vi "main OP300.vi"() -> ()   [LabVIEW 2020]
uses:
  <vilib>/Sylvain.lib/02 SLIM ZEN WS 500/SubVi/FGV.ctl
  SubVI/CheminDeBase.vi
  SubVI/OP300ZP_state.ctl
  OP500/VG/VG_progressBar.vi
  VG/IS30%.vi
  VG/PN.vi
  VG/R.vi
  SubVI/VG_HYDRAU.vi
  VG/VG_BT3562.vi
  VG/VG_ST5520.vi
  VG/VG_MX5060.vi
panel:
  out "ISO- avant découpage":string
  out "ISO+":string
  out "ISO-":string
  out "progression":dbl(slide) scale=0.0..60.0
  out "N° Révision":u32
  out "Compt":i32
  in  "DERNIER2":bool
  in  "last?":bool
  out "Cluster 2":T1
  out "IS30% ?":bool
  out "Cluster":T1
  out "VISA OUT":T2
  out "PN":string
  out "errout":errorcluster={"status"=TRUE, "code"=0, "source"="PCAN_CHANNEL ILLEGAL"}
  out "errout":errorcluster caption="sortie d'erreur"
  out "STOP":bool
  out "TOP":string
  out "DRAW":picture
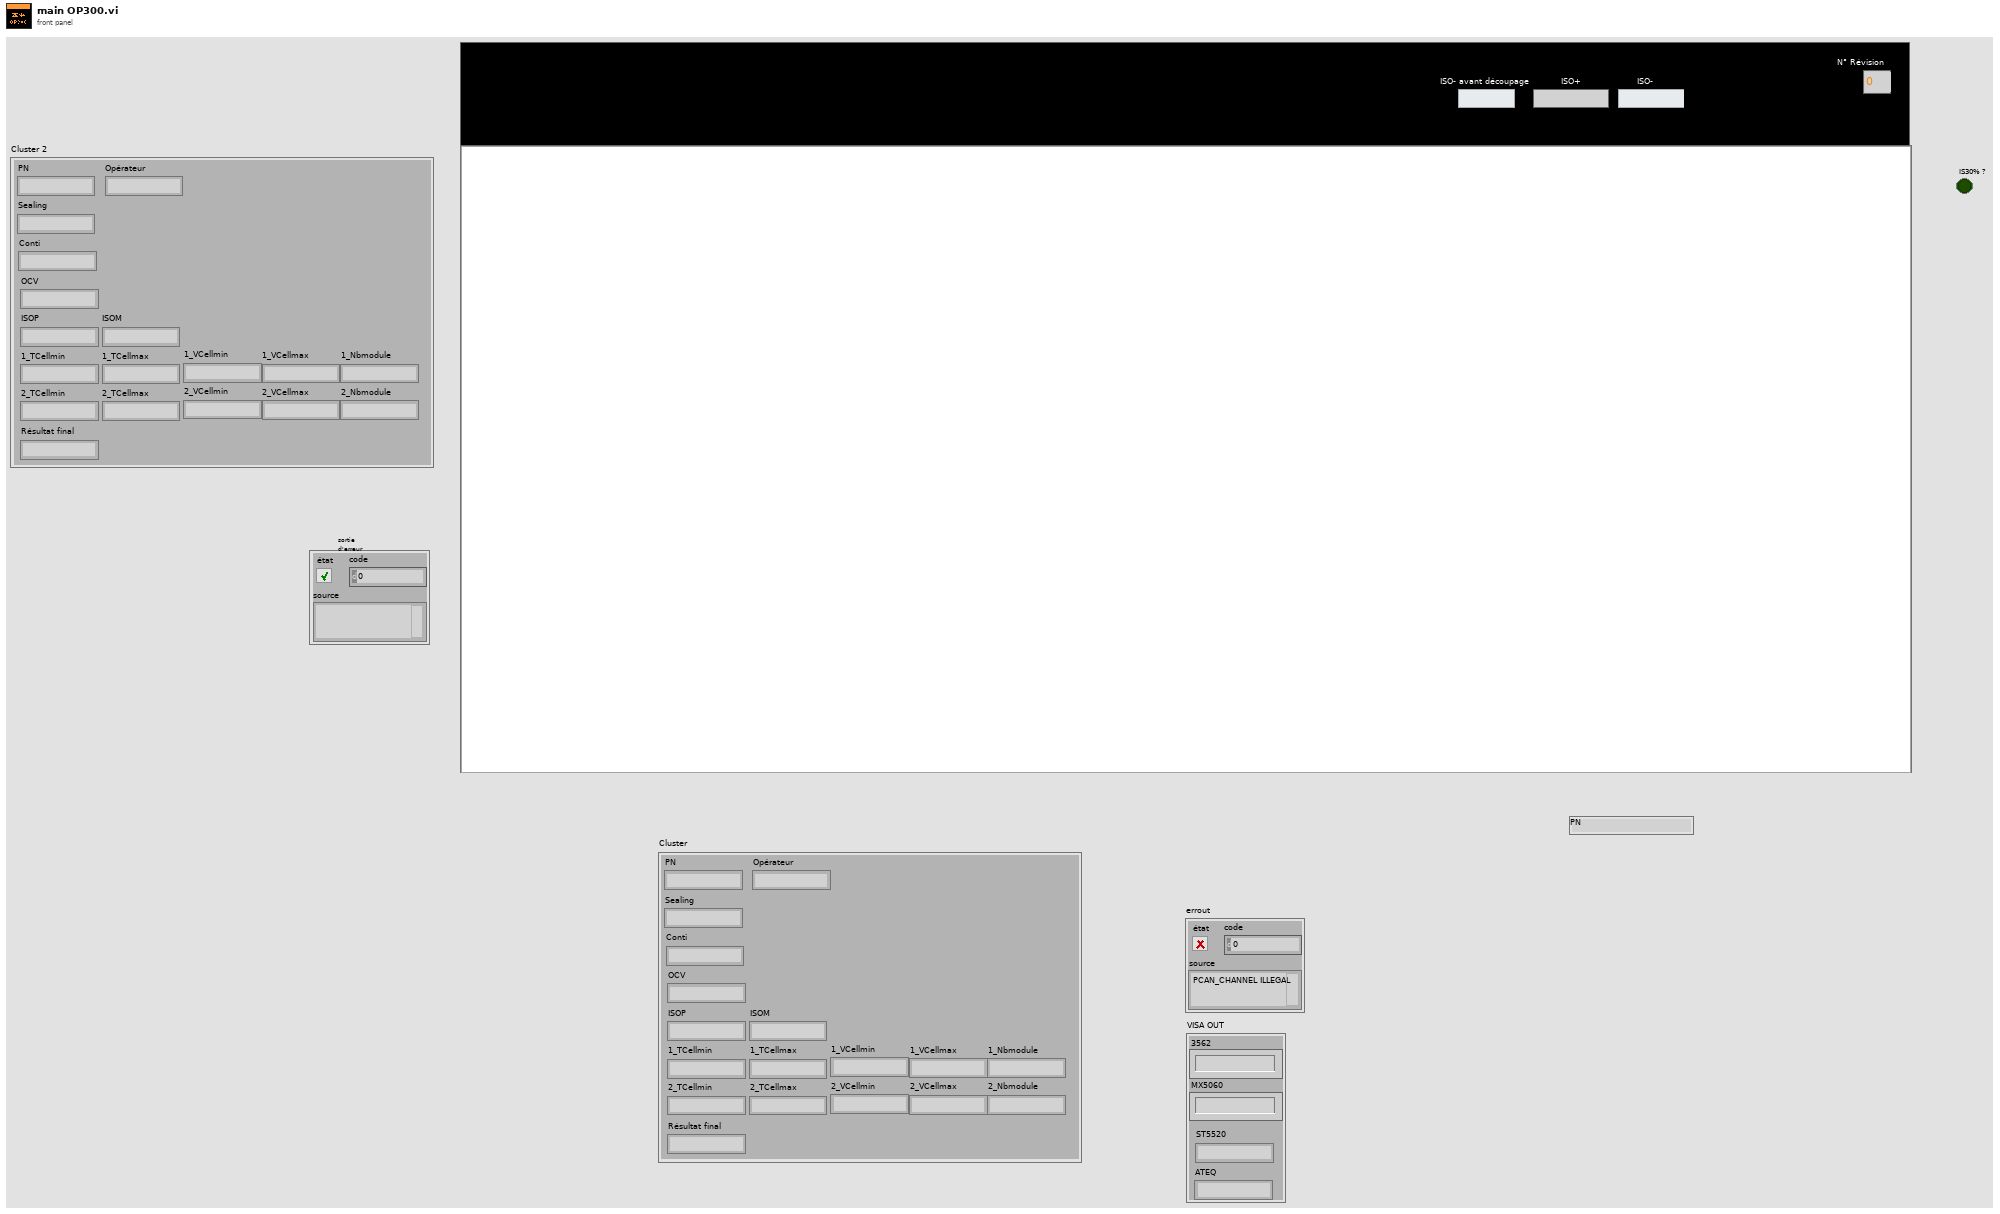
[diagram p1: front panel]
types:
  T1 = cluster{"PN":string, "Opérateur":string, "Sealing":string, "Conti":string, "OCV":string, "ISOP":string, "ISOM":string, "1_TCellmin":string, "1_TCellmax":string, "1_VCellmin":string, "1_VCellmax":string, "1_Nbmodule":string, "2_TCellmin":string, "2_TCellmax":string, "2_VCellmin":string, "2_VCellmax":string, "2_Nbmodule":string, "Résultat final":string}
  T2 = cluster{"3562":string, "MX5060":string, "ST5520":string, "ATEQ":string}
  T3 = cluster{"PN":string, "Sealing":string, "Opérateur":string, "Conti":string, "OCV":string, "ISOP":string, "ISOM":string, "1_TCellmin":string, "1_TCellmax":string, "1_VCellmin":string, "1_VCellmax":string, "1_Nbmodule":string, "2_TCellmin":string, "2_TCellmax":string, "2_VCellmin":string, "2_VCellmax":string, "2_Nbmodule":string, "Résultat final":string}
  T4 = cluster{"3562":string, "MX5060":string, "ST5520":string, "ST5520 2":string}
  T5 = typedef "OP300ZP_state.ctl" = enum16{"Null", "Demarrage", "Init", "Scan", "Montage", "Conti", "OCV", "Iso", "Vpack", "DataDyn", "Dessouter", "DataDyn2", "Demontage", "Crash", "Next", "Hydrau", "Sealing", "Comext"}
  T6 = typedef "FGV.ctl" = enum16{"GET", "SET", "RAZ"}
  T7 = cluster{"1_TCellmin":string, "1_TCellmax":string, "1_VCellmin":string, "1_VCellmax":string, "1_Nbmodule":string, "1_TUsine":string}
  T8 = cluster{"Chaîne":string, "Chaîne":string, "Chaîne":string, "Chaîne":string, "Chaîne":string, "Chaîne":string, "Chaîne":string, "Chaîne 2":string}
  T9 = typedef "imagedata.ctl" = cluster{"image type":i32, "image depth":i32, "image":u8[], "mask":u8[], "colors":u32[], "Rectangle":cluster{"left":i16, "top":i16, "right":i16, "bottom":i16}}
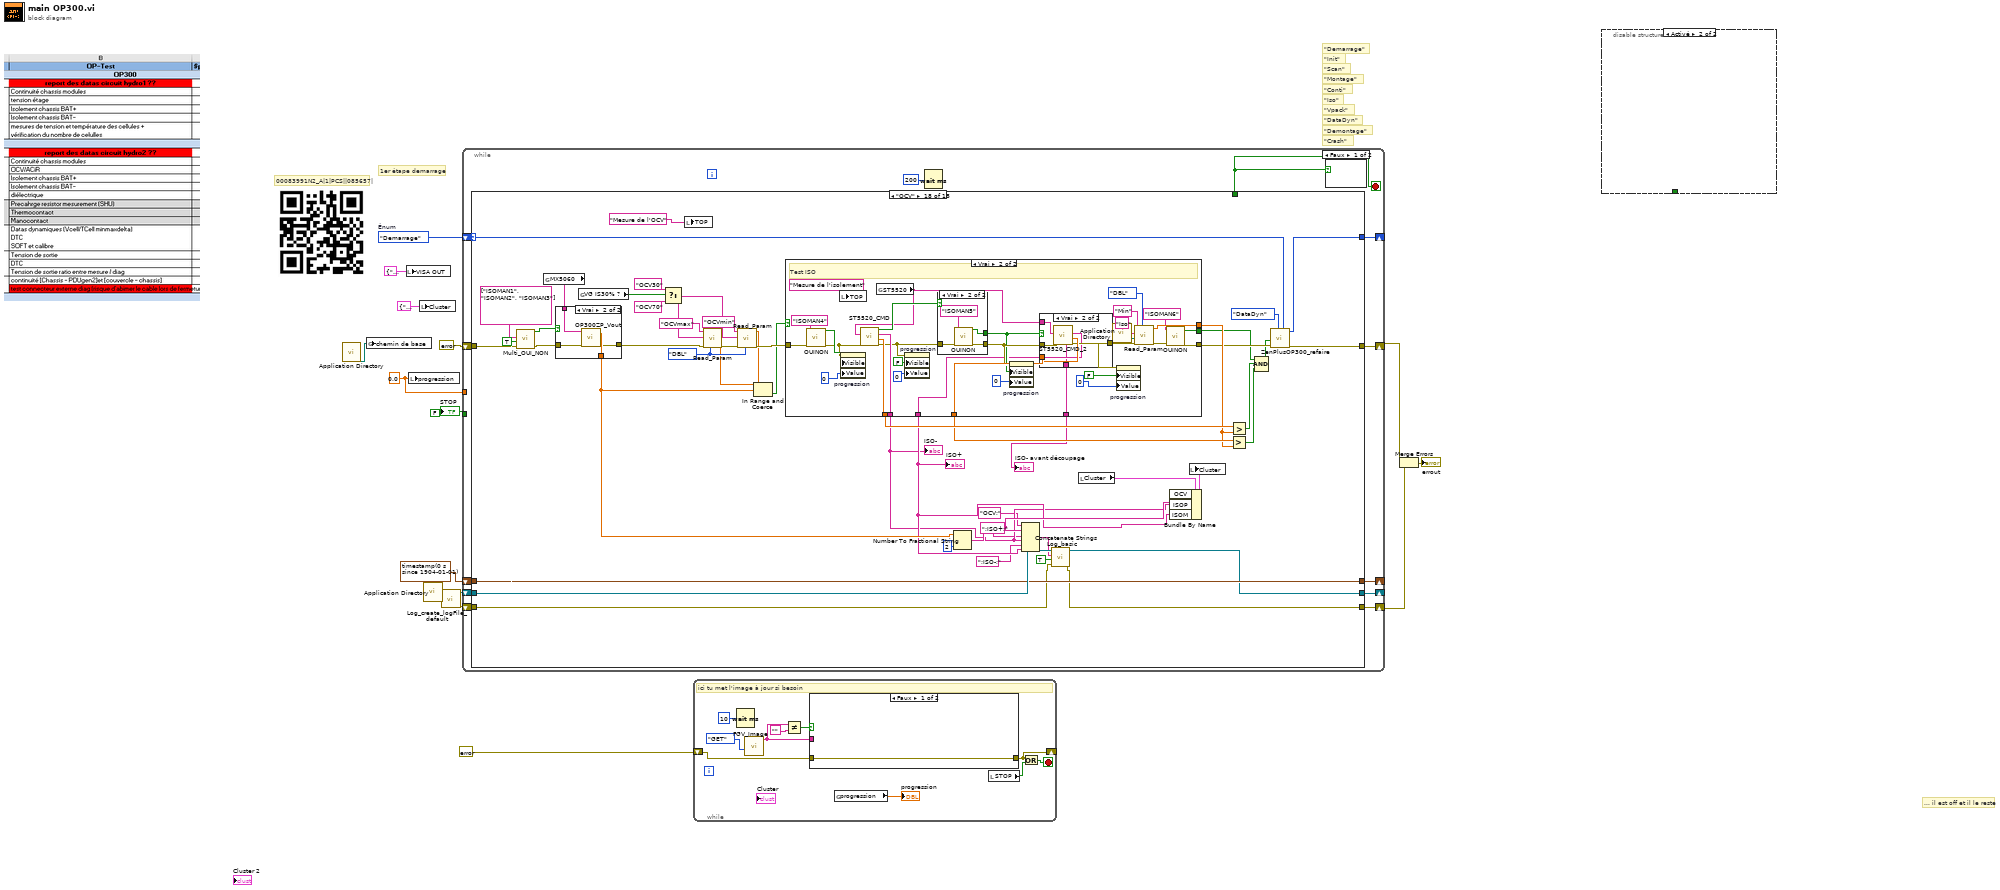
[diagram p0: block diagram]
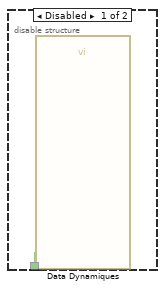
[diagram p2: hidden frame]
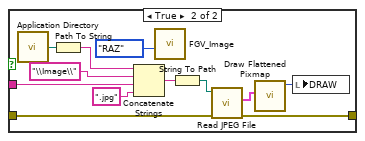
[diagram p3: hidden frame]
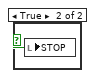
[diagram p4: hidden frame]
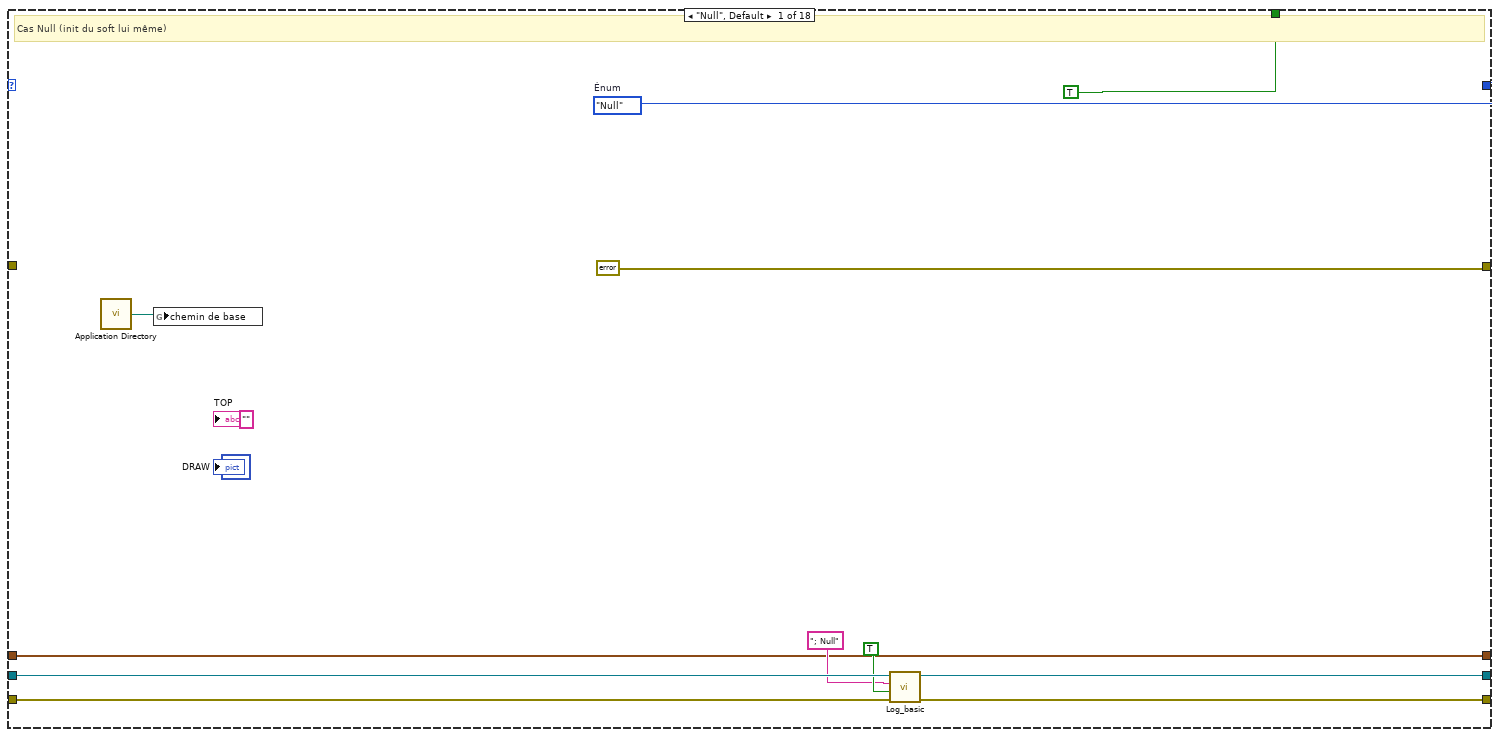
[diagram p5: hidden frame]
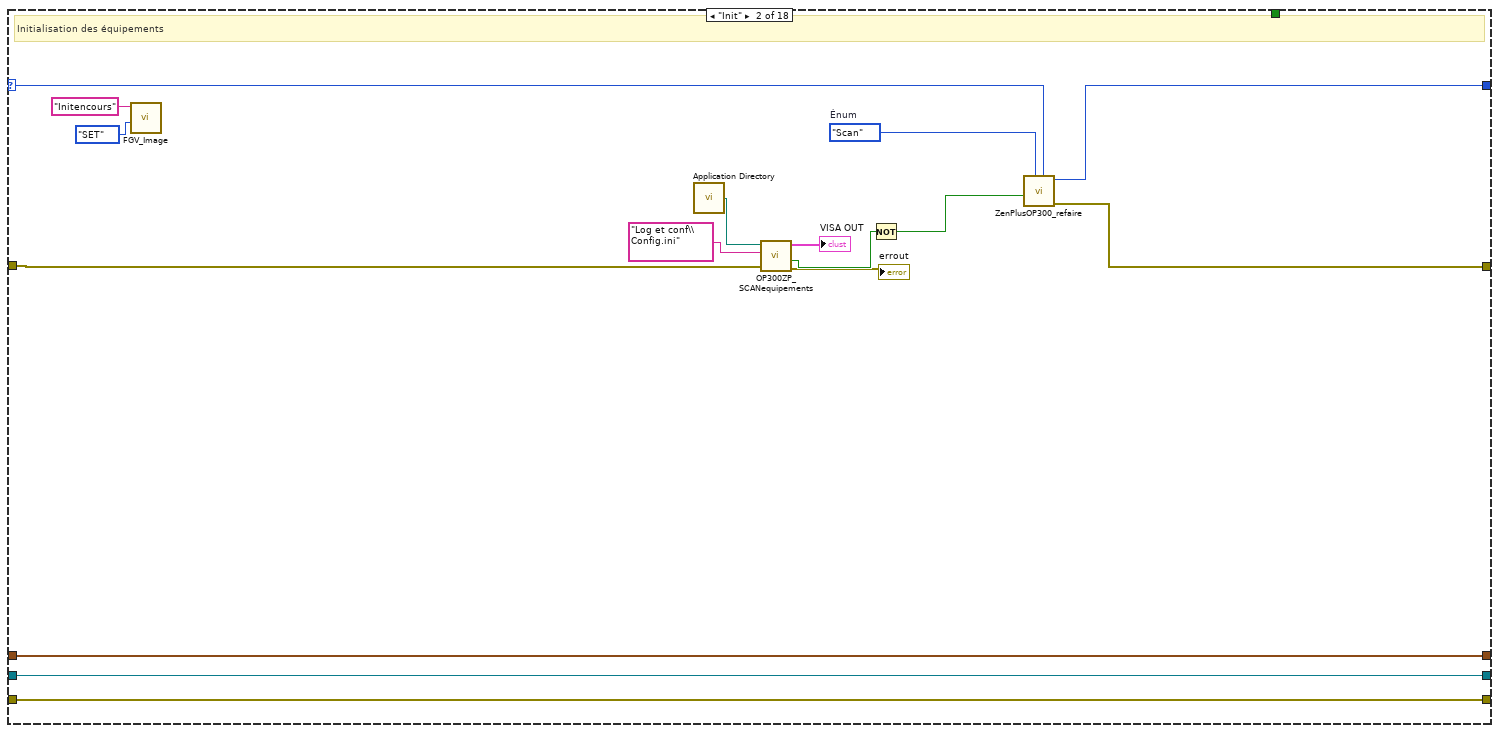
[diagram p6: hidden frame]
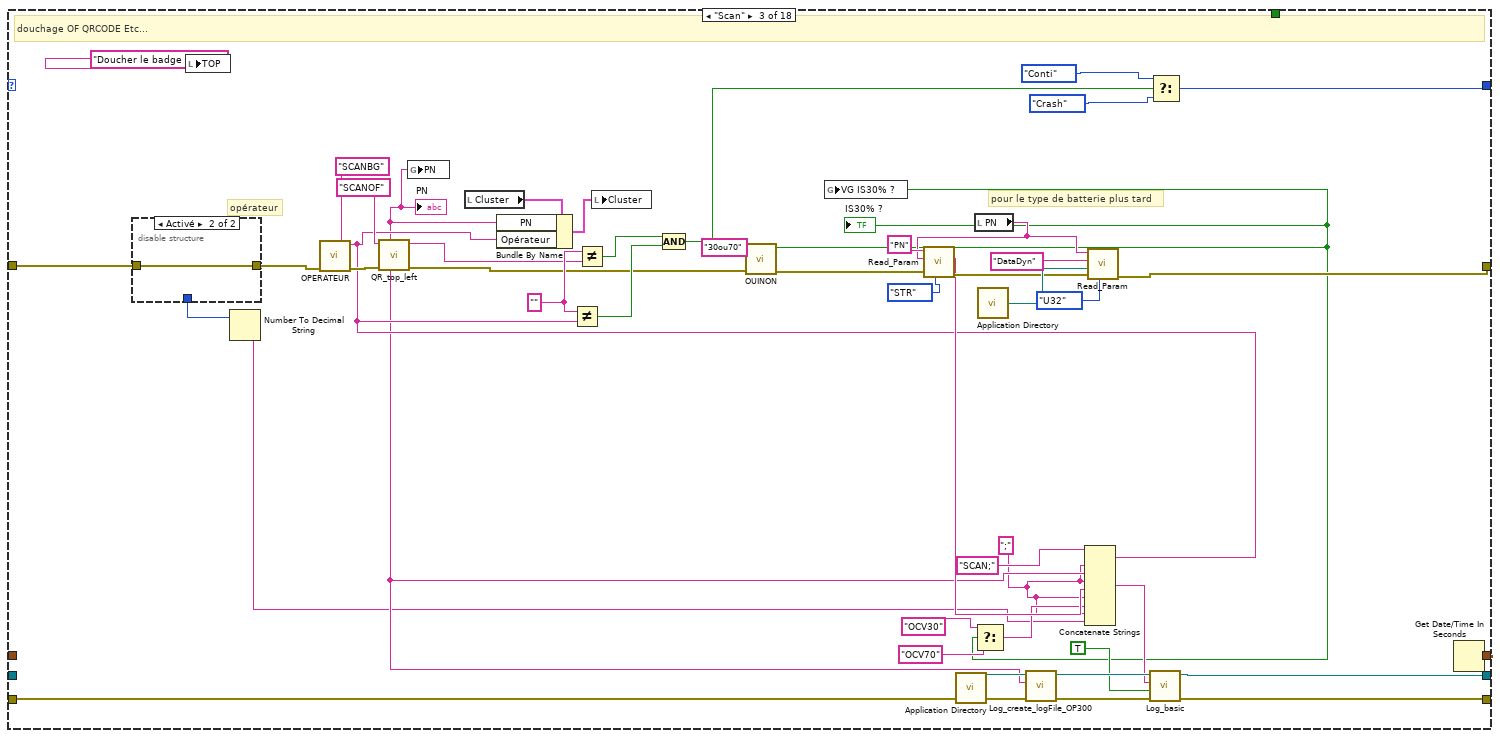
[diagram p7: hidden frame]
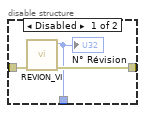
[diagram p8: hidden frame]
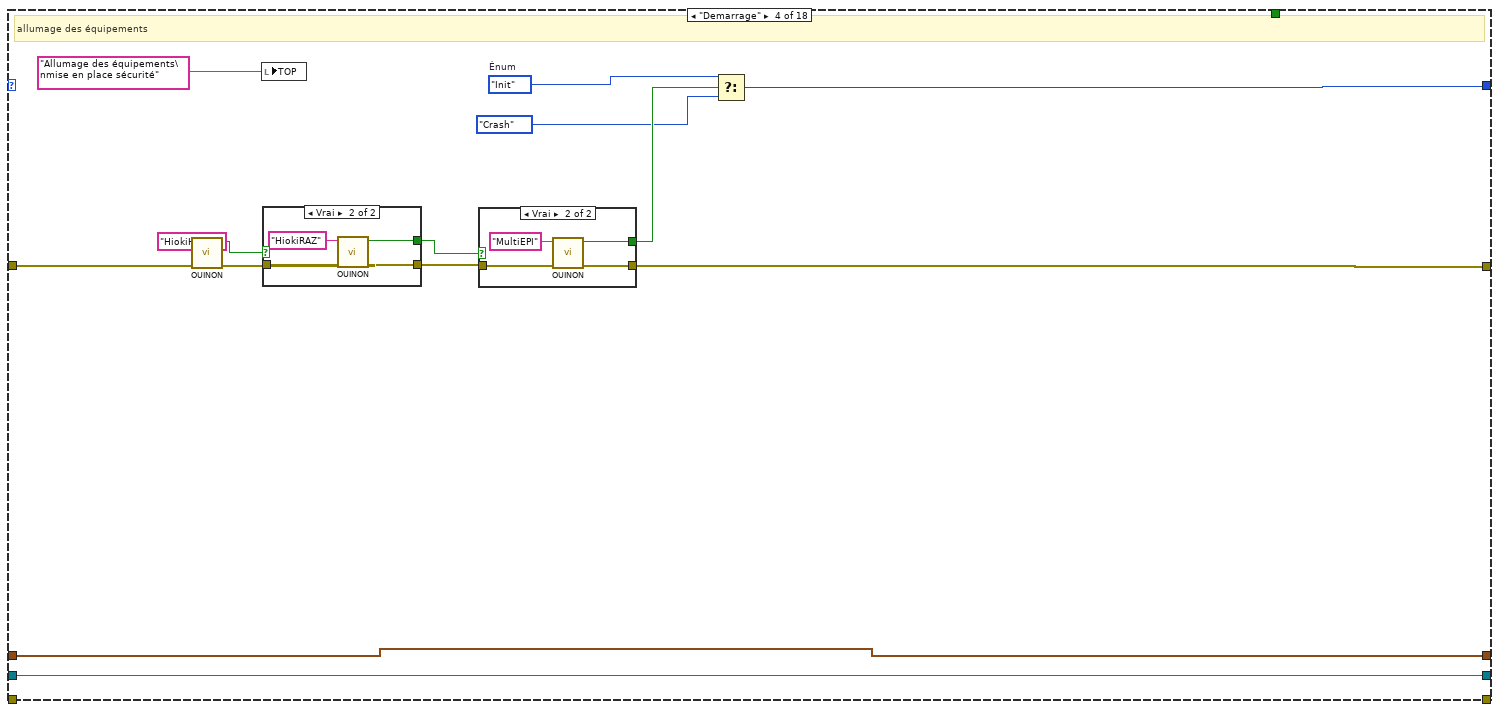
[diagram p9: hidden frame]
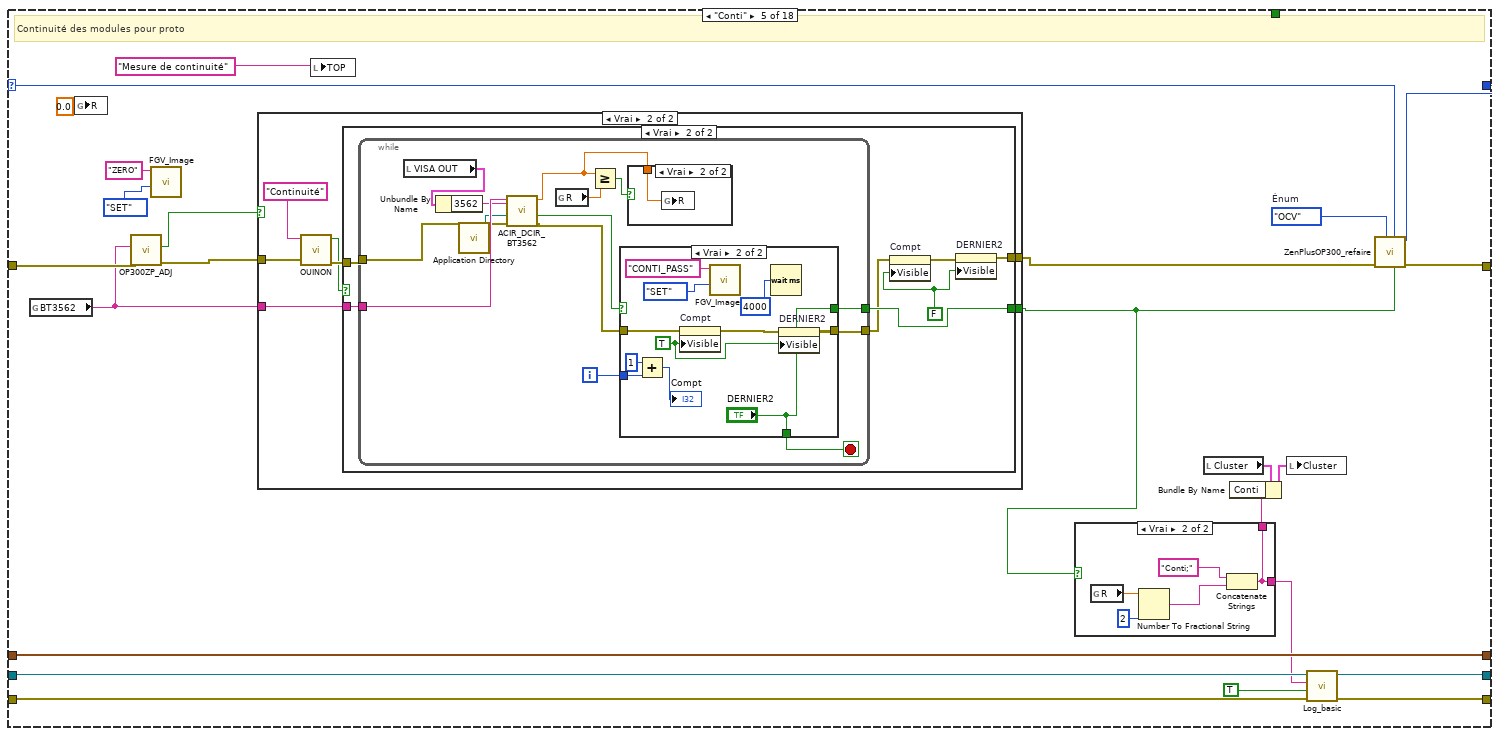
[diagram p12: hidden frame]
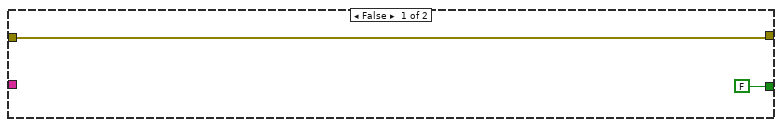
[diagram p13: hidden frame]
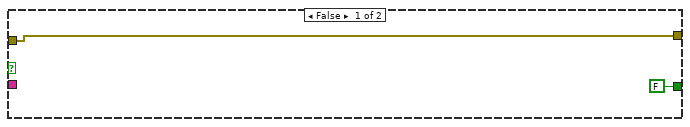
[diagram p14: hidden frame]
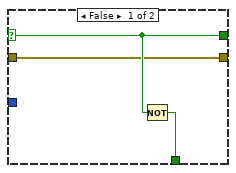
[diagram p15: hidden frame]
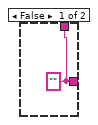
[diagram p17: hidden frame]
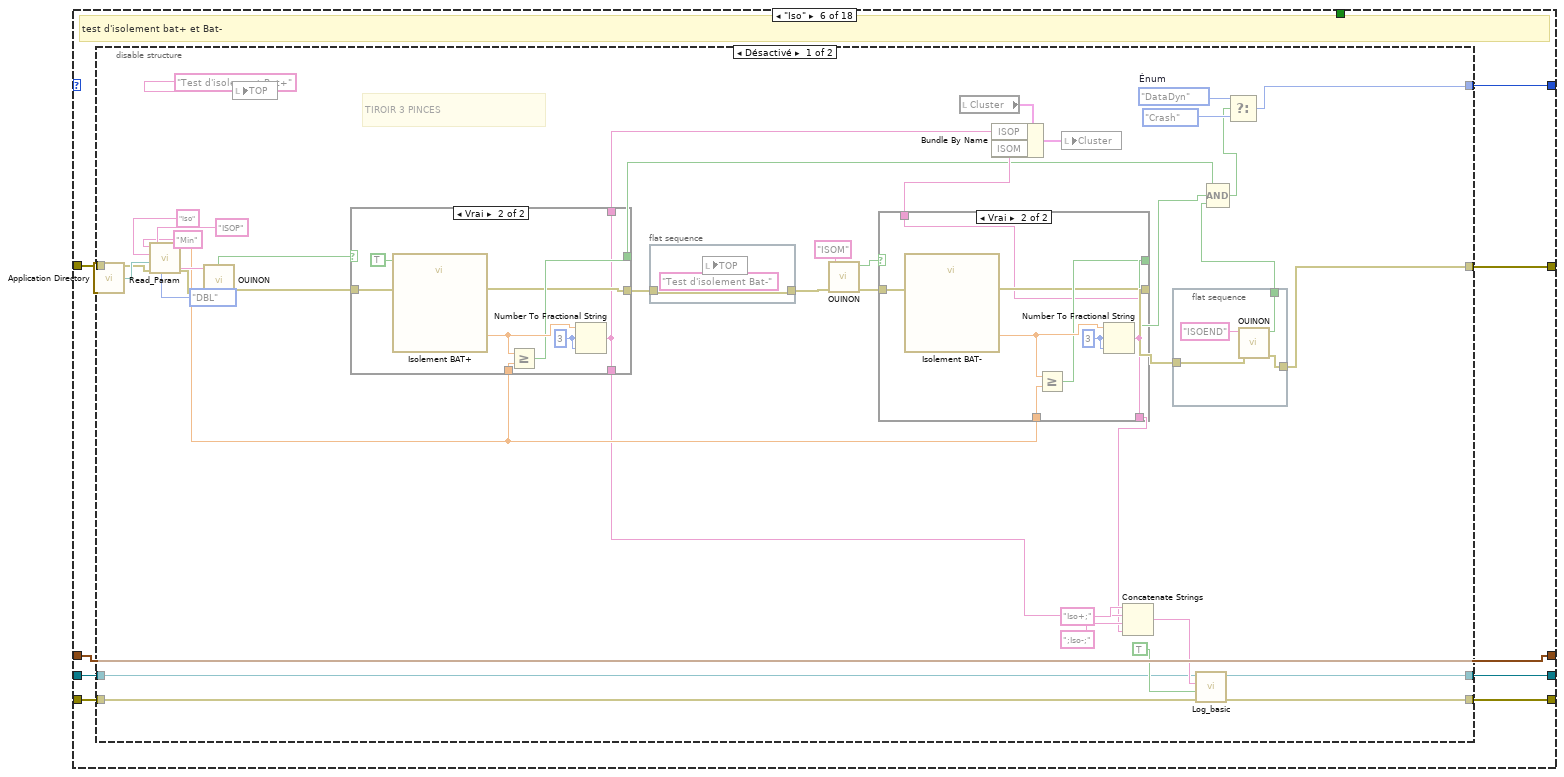
[diagram p18: hidden frame]
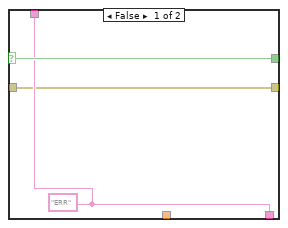
[diagram p19: hidden frame]
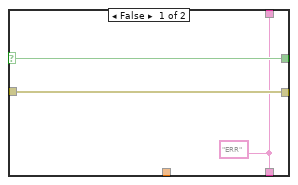
[diagram p20: hidden frame]
diagram:
  w1 = 0.0 ("progression")
  w5 = OP300ZP_state."Demarrage"  # Énum
  w11 = FALSE ("STOP")
  # "00083991N2_A|1|PCS||085657|"
  # "1er étape demarrage"
  # "\"Crash\""
  # "\"Demontage\""
  # "\"DataDyn\""
  # "\"Iso\""
  # "\"Montage\""
  # "\"Scan\""
  # "\"Init\""
  # "\"Demarrage\""
  # "\"Conti\""
  # "\"Vpack\""
  # "... il est off et il le reste"
  n1 = call <vilib>:"Application Directory.vi"() -> ("Application Directory"=w10:path)
  n2 = global write "CheminDeBase.vi" "chemin de base"(w10) -> ()
  n3 = local write "VISA OUT"(T4 {"3562"="", "MX5060"="", "ST5520"="", "ST5520 2"=""} ("VISA OUT")) -> ()
  n4 = local write "progression"(w1) -> ()
  n5 = local write "Cluster"(T3 {"PN"="0", "Sealing"="0", "Opérateur"="0", "Conti"="0", "OCV"="0", "ISOP"="0", "ISOM"="0", "1_TCellmin"="0", "1_TCellmax"="0", "1_VCellmin"="0", "1_VCellmax"="0", "1_Nbmodule"="0", "2_TCellmin"="0", "2_TCellmax"="0", "2_VCellmin"="0", "2_VCellmax"="0", "2_Nbmodule"="0", "Résultat final"="0"} ("Cluster")) -> ()
  n6 = call <vilib>:"Application Directory.vi"() -> ("Application Directory"=w8:path)
  n7 = call <vilib>:"Log_create_logFile_default.vi"("appdir"=w8) -> ("errout"=w9:errorcluster, "Fichier à flux d'octets en sortie"=w12:refnum<file>)  [unwired: 9 in]
  n8 = while {
    shift-right: [w26] -> w14
    shift-left: errorcluster {"status"=FALSE, "code"=0, "source"=""} ("error out") -> [w17]
    shift-right: [w16] -> _
    shift-left: w5 -> [w20]
    shift-right: [w22] -> w13
    shift-left: w9 -> [w25]
    shift-right: [w23] -> _
    shift-left: w12 -> [w24]
    tunnel: w11 -> [_]
    shift-right: [w18] -> _
    shift-left: timestamp(0 s since 1904-01-01) ("seconds since 1Jan1904") -> [w19]
    tunnel: w1 -> [_]
    stop <- w21 stop-if-true
    n9 = case shown="\"OCV\"" w20 {
      selector: w20 -> [_ w53 _ _ w153 _ _ w360 _ w433 _ _ _ _ _ w633 w668 w758]
      tunnel: w17 -> [_ w43 w62 w122 w141 w214 w302 w358 w380 w400 w453 w462 w487 w507 w541 w644 w666 w755]
      tunnel: [errorcluster {"status"=FALSE, "code"=0, "source"=""} ("errin") w54 w86 w121 w154 w215 w306 w359 w387 w395 w452 w461 w487 w505 w544 w631 w667 w763] -> w26
      tunnel: w25 -> [w37 w57 w102 _ w159 w219 w311 w364 w379 w430 w450 w464 w490 w530 w547 w639 w672 w766]
      tunnel: w24 -> [w38 w56 _ w123 w158 w218 w310 w365 w377 w432 w451 w465 w491 w531 w546 w637 w671 w768]
      tunnel: [w35 w56 w104 w123 w157 w217 w309 w362 w377 w428 w451 w465 _ _ w545 w636 w670 w764] -> w23
      tunnel: [w36 w57 w105 _ w156 w220 w308 w363 w379 w429 w450 w464 w480 w523 w542 w638 w669 w765] -> w22
      tunnel: [TRUE _ _ _ _ _ _ _ _ _ _ FALSE w492 _ _ _ _ _] -> w21
      tunnel: w19 -> [w31 w55 _ w120 w155 w216 w289 w361 w378 w431 w449 w460 _ _ w543 w635 w664 w767]
      tunnel: [w31 w55 w93 w120 w155 w216 w289 w361 w378 w431 w449 w460 _ _ w543 w635 w665 w767] -> w18
      tunnel: [w29 w44 w65 w110 w145 w213 w287 w323 w376 w403 w444 w455 OP300ZP_state."Crash" w502 w540 w632 w663 w757] -> w16
      frame "Null", Default {
        w29 = OP300ZP_state."Null"  # Énum
        # "Cas Null (init du soft lui même)"
        n10 = call <vilib>:"Application Directory.vi"() -> ("Application Directory"=w41:path)
        n11 = global write "CheminDeBase.vi" "chemin de base"(w41) -> ()
        n12 = call <vilib>:"Log_basic.vi"("errin"=w37, "date?"=TRUE, "chaîne"="; Null", "in"=w38) -> ("sortie d'erreur"=w36:errorcluster, "refnum en sortie"=w35:refnum<file>)  [unwired: 6 in]
        "DRAW" <- picture data[5B] ("DRAW")
        "TOP" <- "" ("TOP")
      }
      frame "Init" {
        w48 = OP300ZP_state."Scan"  # Énum
        # "Initialisation des équipements"
        n13 = call <vilib>:"FGV_Image.vi"("Énum"=FGV."SET", "IN"="Initencours") -> ()  [unwired: 9 in, 1 out]
        n14 = call <vilib>:"Application Directory.vi"() -> ("Application Directory"=w45:path)
        n15 = call "OP300ZP_SCANequipements.vi"("Errin"=w43, "Chaîne"="Log et conf\\Config.ini", "pathin"=w45) -> ("ERROUT"=→"errout":errorcluster, "KO?"=w49:bool, "VISA OUT"=→"VISA OUT":T2)  [unwired: 6 in]
        n16 = Not(x=w49) -> (.not. x?=w50:bool)
        n17 = call "ZenPlusOP300_refaire.vi"("refaire"=w53, "casOK"=w48, "test ok ?"=w50) -> ("errout"=w54:errorcluster, "Next"=w44:T5)  [unwired: 7 in]
      }
      frame "Scan" {
        w58 = ";" ("chaîne")
        w96 = "" ("x")
        # "pour le type de batterie plus tard"
        # "opérateur"
        # "douchage OF QRCODE Etc..."
        n18 = disable-structure shown="Activé" {
          disable-tunnel: w62 -> [w108 w109]
          disable-tunnel: [w107 w109] -> w61
          disable-tunnel: [w106 _] -> w60
          frame Disabled {
            n19 = call "REVION_VI.vi"("ERRIN"=w108) -> ("ERROUT"=w107:errorcluster, "N° Révision"=w106:u32)  [unwired: 9 in]
            "N° Révision" <- w106
          }
          frame Enabled {
          }
        }
        n20 = local write "TOP"("Doucher le badge et l'OF" ("TOP")) -> ()
        n21 = Number To Decimal String(number=w60) -> (decimal integer string=w59:string)  [unwired: 1 in]
        n22 = call <vilib>:"OPERATEUR.vi"("errin"=w61, "IN"="SCANBG") -> ("error out"=w92:errorcluster, "Dataout"=w73:string)  [unwired: 8 in]
        n23 = call <vilib>:"QR_top_left.vi"("errin"=w92, "image"="SCANOF") -> ("error out"=w63:errorcluster, "Réponse"=w90:string, "SN"=w64:string, "PN"=w66:string)  [unwired: 5 in, 1 out]
        "PN" <- w66
        n24 = global write "PN.vi" "PN"(w66) -> ()
        n25 = local read "Cluster"() -> (w75:T1)
        n26 = Bundle By Name(cluster=w75, "PN"=w66, "Opérateur"=w73) -> (w74:T1)
        n27 = Not Equal?(x=w96, y=w73) -> (x != y?=w94:bool)
        n28 = Not Equal?(x=w96, y=w90) -> (x != y?=w95:bool)
        n29 = local write "Cluster"(w74) -> ()
        n30 = Compound Arithmetic op=AND ("Opérateur arithmétique")(w95, w94) -> (w79:bool)
        n31 = call <vilib>:"OUINON.vi"("errin"=w63, "image"="30ou70") -> ("error out"=w71:errorcluster, "OUI/NON"=w67:bool)  [unwired: 8 in]
        "IS30% ?" <- w67
        n32 = global write "IS30%.vi" "VG IS30% ?"(w67) -> ()
        n33 = call <vilib>:"Application Directory.vi"() -> ("Application Directory"=w103:path)
        n34 = local read "PN"() -> (w82:string)
        n35 = call "Read_Param.vi"("Énum"=enum16{"STR", "DBL", "U32"}."STR", "errin"=w71, "section"=w82, "key"="PN") -> ("error out"=w85:errorcluster, "str"=w81:string)  [unwired: 3 in, 3 out]
        n36 = Select ("Sélectionner")(t="OCV30" ("section"), s=w67, f="OCV70" ("section")) -> (s? t:f=w68:string)
        n37 = call <vilib>:"Application Directory.vi"() -> ("Application Directory"=w89:path)
        n38 = call "Log_create_logFile_OP300.vi"("errin"=w102, "toute l'expression"=w64, "Application Directory"=w103) -> ("sortie d'erreur"=w100:errorcluster, "Fichier à flux d'octets en sortie"=w101:refnum<file>)  [unwired: 7 in]
        n39 = Concatenate Strings("SCAN;" ("chaîne"), w73, w58, w64, w58, w81, w58, w68, w58, w59) -> (w98:string)
        n40 = call "Read_Param.vi"("Énum"=enum16{"STR", "DBL", "U32"}."U32", "errin"=w85, 9:w89, "section"="DataDyn", "key"=w82) -> ("error out"=w86:errorcluster)  [unwired: 2 in, 4 out]
        n41 = call <vilib>:"Log_basic.vi"("errin"=w100, "date?"=TRUE, "chaîne"=w98, "in"=w101) -> ("sortie d'erreur"=w105:errorcluster, "refnum en sortie"=w104:refnum<file>)  [unwired: 6 in]
        n42 = Select ("Sélectionner")(t=OP300ZP_state."Conti" ("Énum"), s=w79, f=OP300ZP_state."Crash" ("cas faux")) -> (s? t:f=w65:T5)
        n43 = Get Date/Time In Seconds() -> (seconds since 1Jan1904=w93:timestamp)
      }
      frame "Demarrage" {
        w112 = OP300ZP_state."Init"  # Énum
        # "allumage des équipements"
        n44 = call <vilib>:"OUINON.vi"("errin"=w122, "image"="HiokiHypot") -> ("error out"=w118:errorcluster, "OUI/NON"=w115:bool)  [unwired: 8 in]
        n45 = local write "TOP"("Allumage des équipements\nmise en place sécurité" ("TOP")) -> ()
        n46 = case shown="Vrai" w115 {
          selector: w115 -> [w125 _]
          tunnel: [w125 w129] -> w116
          tunnel: [w124 w128] -> w117
          tunnel: w118 -> [w124 w126]
          frame False {
          }
          frame True {
            n47 = call <vilib>:"OUINON.vi"("errin"=w126, "image"="HiokiRAZ" ("IN")) -> ("error out"=w128:errorcluster, "OUI/NON"=w129:bool)  [unwired: 8 in]
          }
        }
        n48 = case shown="Vrai" w116 {
          selector: w116 -> [w131 _]
          tunnel: [w131 w135] -> w113
          tunnel: [w130 w134] -> w121
          tunnel: w117 -> [w130 w132]
          frame False {
          }
          frame True {
            n49 = call <vilib>:"OUINON.vi"("errin"=w132, "image"="MultiEPI" ("IN")) -> ("error out"=w134:errorcluster, "OUI/NON"=w135:bool)  [unwired: 8 in]
          }
        }
        n50 = Select ("Sélectionner")(t=w112, s=w113, f=OP300ZP_state."Crash" ("cas faux")) -> (s? t:f=w110:T5)
      }
      frame "Conti" {
        w149 = OP300ZP_state."OCV"  # Énum
        # "Continuité des modules pour proto"
        n51 = global read "VG_BT3562.vi" "BT3562"() -> (w137:string)
        n52 = global write "R.vi" "R"(0.0 ("R")) -> ()
        n53 = call "OP300ZP_ADJ.vi"("errin"=w141, "BT3562A"=w137) -> ("errout"=w140:errorcluster, "ADJ?"=w138:bool)  [unwired: 8 in]
        n54 = call <vilib>:"FGV_Image.vi"("Énum"=FGV."SET", "IN"="ZERO") -> ()  [unwired: 9 in, 1 out]
        n55 = case shown="Vrai" w138 {
          tunnel: [FALSE ("DERNIER2") w168] -> w146
          tunnel: [w161 w167] -> w147
          tunnel: w140 -> [w161 w164]
          tunnel: w137 -> [_ w166]
          frame False {
          }
          frame True {
            n56 = call <vilib>:"OUINON.vi"("errin"=w164, "image"="Continuité" ("IN")) -> ("error out"=w163:errorcluster, "OUI/NON"=w162:bool)  [unwired: 8 in]
            n57 = case shown="Vrai" w162 {
              tunnel: [FALSE ("DERNIER2") w177] -> w168
              tunnel: [w170 w176] -> w167
              tunnel: w166 -> [_ w172]
              tunnel: w163 -> [w170 w171]
              frame False {
              }
              frame True {
                w173 = FALSE ("Visible")
                n58 = while {
                  tunnel: w172 -> [w191]
                  tunnel: w171 -> [w190]
                  tunnel: [w187] -> w175
                  tunnel: [w182] -> w177
                  i -> [w186]
                  stop <- w181 stop-if-true
                  n59 = local read "VISA OUT"() -> (w179:T2)
                  n60 = Unbundle By Name(w179) -> ("3562"=w178:string)
                  n61 = call <vilib>:"Application Directory.vi"() -> ("Application Directory"=w189:path)
                  n62 = call <userlib>:"ACIR_DCIR_BT3562.vi"("errin"=w190, "chemin de base"=w189, "section"=w178, "VISAin"=w191) -> ("errout"=w180:errorcluster, "R pass"=w188:bool, "R Out float"=w183:dbl)  [unwired: 1 in, 4 out]
                  n63 = global read "R.vi" "R"() -> (w185:dbl)
                  n64 = Greater Or Equal?(x=w183, y=w185) -> (x >= y?=w184:bool)
                  n65 = case shown="Vrai" w188 {
                    selector: w188 -> [w194 _]
                    tunnel: w180 -> [w192 w201]
                    tunnel: [w192 w197] -> w187
                    tunnel: [w193 "DERNIER2"] -> w181
                    tunnel: w186 -> [_ w203]
                    tunnel: [w194 "DERNIER2"] -> w182
                    frame False {
                      n66 = Not(x=w194) -> (.not. x?=w193:bool)
                    }
                    frame True {
                      w195 = TRUE ("Visible")
                      n67 = Add(x=1, y=w203) -> (x+y=→"Compt":i32)
                      n68 = property on="Compt" class="NumNb (strict)"(error in=w201, "Visible"=w195) -> (error out=w198:errorcluster)  [unwired: 1 in, 1 out]
                      n69 = call <vilib>:"FGV_Image.vi"("Énum"=FGV."SET", "IN"="CONTI_PASS") -> ()  [unwired: 9 in, 1 out]
                      n70 = Wait (ms)(milliseconds to wait=u32 4000 ("attente (ms)")) -> ()  [unwired: 1 out]
                      n71 = property on="DERNIER2" class="Bool"(error in=w198, "Visible"=w195) -> (error out=w197:errorcluster)  [unwired: 1 in, 1 out]
                    }
                  }
                  n72 = case shown="Vrai" w184 {
                    tunnel: w183 -> [_ w206]
                    frame False {
                    }
                    frame True {
                      n73 = global write "R.vi" "R"(w206) -> ()
                    }
                  }
                }
                n74 = property on="Compt" class="NumNb (strict)"(error in=w175, "Visible"=w173) -> (error out=w174:errorcluster)  [unwired: 1 in, 1 out]
                n75 = property on="DERNIER2" class="Bool"(error in=w174, "Visible"=w173) -> (error out=w176:errorcluster)  [unwired: 1 in, 1 out]
              }
            }
          }
        }
        n76 = local write "TOP"("Mesure de continuité" ("TOP")) -> ()
        n77 = case shown="Vrai" w146 {
          tunnel: [w207 w208] -> w152
          tunnel: [w207 w208] -> w142
          frame False {
            w207 = ""
          }
          frame True {
            n78 = global read "R.vi" "R"() -> (w211:dbl)
            n79 = Number To Fractional String(number=w211, precision (6)=i16 2 ("précision (6)")) -> (F-format string=w210:string)  [unwired: 2 in]
            n80 = Concatenate Strings("Conti;" ("chaîne"), w210) -> (w208:string)
          }
        }
        n81 = local read "Cluster"() -> (w144:T1)
        n82 = Bundle By Name(cluster=w144, "Conti"=w142) -> (w143:T1)
        n83 = local write "Cluster"(w143) -> ()
        n84 = call <vilib>:"Log_basic.vi"("errin"=w159, "date?"=TRUE, "chaîne"=w152, "in"=w158) -> ("sortie d'erreur"=w156:errorcluster, "refnum en sortie"=w157:refnum<file>)  [unwired: 6 in]
        n85 = call "ZenPlusOP300_refaire.vi"("refaire"=w153, "casOK"=w149, "errin"=w147, "test ok ?"=w146) -> ("errout"=w154:errorcluster, "Next"=w145:T5)  [unwired: 6 in]
      }
      frame "Iso" {
        # "test d'isolement bat+ et Bat-"
        n86 = disable-structure shown="Désactivé" {
          disable-tunnel: [w247 _] -> w220
          disable-tunnel: w219 -> [w246 _]
          disable-tunnel: w218 -> [w245 _]
          disable-tunnel: [w244 _] -> w217
          disable-tunnel: [w234 _] -> w215
          disable-tunnel: w214 -> [w222 _]
          disable-tunnel: [w221 _] -> w213
          frame Disabled {
            w240 = OP300ZP_state."DataDyn"  # Énum
            # "TIROIR 3 PINCES"
            n87 = call <vilib>:"Application Directory.vi"() -> ("Application Directory"=w255:path)
            n88 = call "Read_Param.vi"("Énum"=enum16{"STR", "DBL", "U32"}."DBL", "errin"=w222, 9:w255, "section"="Iso", "key"="Min") -> ("error out"=w252:errorcluster, "dbl"=w249:dbl)  [unwired: 2 in, 3 out]
            n89 = call <vilib>:"OUINON.vi"("errin"=w252, "image"="ISOP" ("IN")) -> ("error out"=w227:errorcluster, "OUI/NON"=w228:bool)  [unwired: 8 in]
            n90 = local write "TOP"("Test d'isolement Bat+" ("TOP")) -> ()
            n91 = case shown="Vrai" w228 {
              selector: w228 -> [w277 _]
              tunnel: w227 -> [w278 w286]
              tunnel: [w278 w281] -> w225
              tunnel: [w276 w280] -> w242
              tunnel: [w277 w282] -> w232
              tunnel: w249 -> [_ w284]
              tunnel: [w276 w280] -> w236
              frame False {
                w276 = "ERR"
              }
              frame True {
                w285 = i16 3 ("largeur (-)")
                n92 = call "Isolement BAT+"("Enable"=TRUE, "error in (no error)"=w286) -> ("ISOP"=w283:dbl, "error out"=w281:errorcluster)  [unwired: 15 in, 1 out]
                n93 = Greater Or Equal?(x=w283, y=w284) -> (x >= y?=w282:bool)
                n94 = Number To Fractional String(number=w283, width (-)=w285, precision (6)=w285) -> (F-format string=w280:string)  [unwired: 1 in]
              }
            }
            n95 = flat-sequence {
              tunnel: w225 -> [w260]
              tunnel: [w260] -> w224
              frame #0 {
                n96 = local write "TOP"("Test d'isolement Bat-" ("TOP")) -> ()
              }
            }
            n97 = call <vilib>:"OUINON.vi"("errin"=w224, "image"="ISOM" ("IN")) -> ("error out"=w226:errorcluster, "OUI/NON"=w250:bool)  [unwired: 8 in]
            n98 = case shown="Vrai" w250 {
              selector: w250 -> [w268 _]
              tunnel: [w266 w271] -> w233
              tunnel: [w267 w270] -> w241
              tunnel: [w268 w272] -> w231
              tunnel: w249 -> [_ w274]
              tunnel: [w267 w270] -> w235
              tunnel: w226 -> [w266 w269]
              frame False {
                w267 = "ERR"
              }
              frame True {
                w275 = i16 3 ("largeur (-)")
                n99 = call "Isolement BAT-"("error in (no error)"=w269) -> ("ISOM"=w273:dbl, "error out"=w271:errorcluster)  [unwired: 16 in, 1 out]
                n100 = Greater Or Equal?(x=w273, y=w274) -> (x >= y?=w272:bool)
                n101 = Number To Fractional String(number=w273, width (-)=w275, precision (6)=w275) -> (F-format string=w270:string)  [unwired: 1 in]
              }
            }
            n102 = local read "Cluster"() -> (w238:T1)
            n103 = Bundle By Name(cluster=w238, "ISOP"=w236, "ISOM"=w235) -> (w237:T1)
            n104 = local write "Cluster"(w237) -> ()
            n105 = Concatenate Strings("Iso+;" ("chaîne"), w242, ";Iso-;" ("chaîne"), w241) -> (w258:string)
            n106 = flat-sequence {
              tunnel: [w263] -> w234
              tunnel: w233 -> [w264]
              tunnel: [w262] -> w230
              frame #0 {
                n107 = call <vilib>:"OUINON.vi"("errin"=w264, "image"="ISOEND") -> ("error out"=w263:errorcluster, "OUI/NON"=w262:bool)  [unwired: 8 in]
              }
            }
            n108 = call <vilib>:"Log_basic.vi"("errin"=w246, "date?"=TRUE, "chaîne"=w258, "in"=w245) -> ("sortie d'erreur"=w247:errorcluster, "refnum en sortie"=w244:refnum<file>)  [unwired: 6 in]
            n109 = Compound Arithmetic op=AND ("Opérateur arithmétique")(w232, w231, w230) -> (w229:bool)
            n110 = Select ("Sélectionner")(t=w240, s=w229, f=OP300ZP_state."Crash" ("cas faux")) -> (s? t:f=w221:T5)
          }
          frame Enabled {
          }
        }
      }
      frame "Vpack" {
        w288 = OP300ZP_state."DataDyn"  # Énum
        w297 = enum16{"STR", "DBL", "U32"}."DBL" ("Énum")
        w300 = "Vpack" ("section")
        # "SKIP"
        # "tension du pack en sortie"
        n111 = call <vilib>:"Application Directory.vi"() -> ("Application Directory"=w298:path)
        n112 = call "Read_Param.vi"("Énum"=w297, "errin"=w302, 9:w298, "section"=w300, "key"="Min") -> ("error out"=w303:errorcluster, "dbl"=w295:dbl)  [unwired: 2 in, 3 out]
        n113 = call "Read_Param.vi"("Énum"=w297, "errin"=w303, 9:w298, "section"=w300, "key"="Max") -> ("error out"=w301:errorcluster, "dbl"=w296:dbl)  [unwired: 2 in, 3 out]
        n114 = call <vilib>:"OUINON.vi"("errin"=w301, "image"="Vpack" ("IN")) -> ("error out"=w305:errorcluster, "OUI/NON"=w292:bool)  [unwired: 8 in]
        n115 = case shown="Vrai" w292 {
          selector: w292 -> [w312 _]
          tunnel: w305 -> [w314 w322]
          tunnel: [w314 w319] -> w306
          tunnel: ["ERR" w320] -> w290
          tunnel: [w312 w317] -> w291
          tunnel: w296 -> [_ w315]
          tunnel: w295 -> [_ w316]
          frame False {
          }
          frame True {
            w321 = i16 3 ("largeur (-)")
            n116 = call "Tension de l'étage bas"("error in (no error)"=w322) -> ("Vpack"=w318:dbl, "error out"=w319:errorcluster)  [unwired: 16 in, 1 out]
            n117 = In Range and Coerce(upper limit=w315, x=w318, lower limit=w316) -> (In Range?=w317:bool)  [unwired: 1 out]
            n118 = Number To Fractional String(number=w318, width (-)=w321, precision (6)=w321) -> (F-format string=w320:string)  [unwired: 1 in]
          }
        }
        n119 = call "OP400ZP_prep bdd Vpack.vi"("OCV"=w290) -> ()  [unwired: 10 in, 1 out]
        n120 = Concatenate Strings("Vpack;" ("chaîne"), w290) -> (w293:string)
        n121 = call "OP300ZP_OuCrash.vi"("Booléen"=w291, "in"=w288) -> ("OUT"=w287:T5)  [unwired: 1 in]
        n122 = call <vilib>:"Log_basic.vi"("errin"=w311, "chaîne"=w293, "in"=w310) -> ("sortie d'erreur"=w308:errorcluster, "refnum en sortie"=w309:refnum<file>)  [unwired: 7 in]
      }
      frame "DataDyn" {
        (unwired) "Refaire" ("image")
        # "A supprimer avec nouvelle config ISO SPI"
        # "Divers data du pack"
        n123 = local write "TOP"("Analyse 1 des CMU ..." ("TOP")) -> ()
        n124 = call <vilib>:"FGV_Image.vi"("Énum"=FGV."SET", "IN"="J1ON") -> ("OUT"=w339:string)  [unwired: 9 in]
        n125 = call <vilib>:"OUINON.vi"("errin"=w358, "image"=w339) -> ("error out"=w338:errorcluster)  [unwired: 8 in, 1 out]
        n126 = property on="progression" class="Gliss (strict)"(error in=w338, "Visible"=TRUE, "Value"=u8 0 ("progression")) -> (error out=w345:errorcluster)  [unwired: 1 in, 1 out]
        n127 = flat-sequence {
          tunnel: [w375] -> w354
          tunnel: [w374] -> w353
          tunnel: [w373] -> w352
          tunnel: [w372] -> w351
          tunnel: [w371] -> w350
          tunnel: [w370] -> w349
          tunnel: w345 -> [w369]
          frame #0 {
            n128 = call "SCAN CMU.vi"("errin"=w369, "Nb modules"=i16 16) -> ("errout"=w375:errorcluster, "# température + #tension OK?"=w370:bool, "Vmin"=w374:dbl, "Vmax"=w373:dbl, "Tmin"=w371:dbl, "Tmax"=w372:dbl)  [unwired: 4 out]
            n129 = call <vilib>:"FGV_Image.vi"("Énum"=FGV."SET", "IN"="DataDyn") -> ()  [unwired: 9 in, 1 out]
          }
        }
        n130 = global read "IS30%.vi" "VG IS30% ?"() -> (w324:bool)
        n131 = call "OP400ZP_Test_DataDyn.vi"("Tcell Min (°C)"=w350, "is30%?"=w324, "MCU"=w349, "Tcell Max (°C)"=w351, "Température usine (°C)"=21.0, "errin"=w354, "testname"="Dyn;", "Vcell Min (V)"=w353, "Vcell Max (V)"=w352) -> ("pass"=w325:bool, "datalog"=w357:string, "Cluster"=w333:T7, "errout"=w326:errorcluster)  [unwired: 2 in, 1 out]
        n132 = Unbundle By Name(w333) -> ("1_TCellmin"=w332:string, "1_TCellmax"=w331:string, "1_VCellmin"=w330:string, "1_VCellmax"=w329:string, "1_Nbmodule"=w328:string)
        n133 = local read "Cluster"() -> (w335:T1)
        n134 = Bundle By Name(cluster=w335, "1_TCellmin"=w332, "1_TCellmax"=w331, "1_VCellmin"=w330, "1_VCellmax"=w329, "1_Nbmodule"=w328) -> (w334:T1)
        n135 = call "ZenPlusOP300_refaire.vi"("refaire"=w360, "Pédale"=FALSE, "casOK"=OP300ZP_state."Dessouter" ("Énum"), "errin"=w326, "test ok ?"=w325) -> ("errout"=w327:errorcluster, "Next"=w323:T5)  [unwired: 5 in]
        n136 = call <vilib>:"Log_basic.vi"("errin"=w364, "date?"=TRUE, "chaîne"=w357, "in"=w365) -> ("sortie d'erreur"=w363:errorcluster, "refnum en sortie"=w362:refnum<file>)  [unwired: 6 in]
        n137 = local write "Cluster"(w334) -> ()
        n138 = property on="progression" class="Gliss (strict)"(error in=w327, "Visible"=FALSE, "Value"=u8 0 ("progression")) -> (error out=w359:errorcluster)  [unwired: 1 in, 1 out]
      }
      frame "Dessouter" {
        n139 = local write "TOP"("Prendre le MODOP DESSOUTER" ("TOP")) -> ()
        n140 = call <vilib>:"FGV_Image.vi"("Énum"=FGV."SET", "IN"="Echangeur") -> ("OUT"=w392:string)  [unwired: 9 in]
        n141 = call <vilib>:"OUINON.vi"("errin"=w380, "image"=w392) -> ("error out"=w388:errorcluster, "OUI/NON"=w385:bool)  [unwired: 8 in]
        n142 = call <vilib>:"FGV_Image.vi"("Énum"=FGV."SET", "IN"="DessouterEnd") -> ("OUT"=w391:string)  [unwired: 9 in]
        n143 = call <vilib>:"OUINON.vi"("errin"=w388, "image"=w391) -> ("error out"=w387:errorcluster, "OUI/NON"=w386:bool)  [unwired: 8 in]
        n144 = Compound Arithmetic op=AND(w385, w386) -> (w384:bool)
        n145 = Select(t=OP300ZP_state."DataDyn2" ("Next"), s=w384, f=OP300ZP_state."Crash" ("cas faux")) -> (s? t:f=w376:T5)
      }
      frame "DataDyn2" {
        (unwired) "Refaire" ("image")
        n146 = property on="progression" class="Gliss (strict)"(error in=w400, "Visible"=TRUE, "Value"=u8 0 ("progression")) -> (error out=w399:errorcluster)  [unwired: 1 in, 1 out]
        n147 = local write "TOP"("Analyse 2 des CMU ..." ("TOP")) -> ()
        n148 = flat-sequence {
          tunnel: [w443] -> w406
          tunnel: [w442] -> w425
          tunnel: [w441] -> w424
          tunnel: [w440] -> w423
          tunnel: [w439] -> w422
          tunnel: [w438] -> w421
          tunnel: w399 -> [w437]
          frame #0 {
            n149 = call "SCAN CMU.vi"("errin"=w437, "Nb modules"=i16 16) -> ("errout"=w443:errorcluster, "# température + #tension OK?"=w438:bool, "Vmin"=w442:dbl, "Vmax"=w441:dbl, "Tmin"=w439:dbl, "Tmax"=w440:dbl)  [unwired: 4 out]
            n150 = call <vilib>:"FGV_Image.vi"("Énum"=FGV."SET", "IN"="DataDyn") -> ()  [unwired: 9 in, 1 out]
          }
        }
        n151 = global read "IS30%.vi" "VG IS30% ?"() -> (w404:bool)
        n152 = call "OP400ZP_Test_DataDyn.vi"("Tcell Min (°C)"=w422, "is30%?"=w404, "MCU"=w421, "Tcell Max (°C)"=w423, "Température usine (°C)"=21.0, "errin"=w406, "testname"="Dyn2;", "Vcell Min (V)"=w425, "Vcell Max (V)"=w424) -> ("pass"=w405:bool, "datalog"=w427:string, "StrData"=w409:T8, "errout"=w407:errorcluster)  [unwired: 2 in, 1 out]
        n153 = Unbundle By Name(w409) -> ("Chaîne"=w414:string, "Chaîne"=w413:string, "Chaîne"=w412:string, "Chaîne"=w411:string, "Chaîne"=w410:string)
        n154 = local read "Cluster"() -> (w416:T1)
        n155 = call <vilib>:"Log_basic.vi"("errin"=w430, "date?"=TRUE, "chaîne"=w427, "in"=w432) -> ("sortie d'erreur"=w429:errorcluster, "refnum en sortie"=w428:refnum<file>)  [unwired: 6 in]
        n156 = call "ZenPlusOP300_refaire.vi"("refaire"=w433, "Pédale"=FALSE, "casOK"=OP300ZP_state."Demontage" ("Énum"), "errin"=w407, "test ok ?"=w405) -> ("errout"=w396:errorcluster, "Next"=w403:T5)  [unwired: 5 in]
        n157 = Bundle By Name(cluster=w416, "2_TCellmin"=w414, "2_TCellmax"=w413, "2_VCellmin"=w412, "2_VCellmax"=w411, "2_Nbmodule"=w410) -> (w415:T1)
        n158 = property on="progression" class="Gliss (strict)"(error in=w396, "Visible"=FALSE, "Value"=u8 0 ("progression")) -> (error out=w395:errorcluster)  [unwired: 1 in, 1 out]
        n159 = local write "Cluster"(w415) -> ()
      }
      frame "Montage" {
        w447 = OP300ZP_state."Conti"  # Énum
        # "montage du produit sur le banc"
        n160 = local write "TOP"("Montage du pack" ("TOP")) -> ()
        n161 = call <vilib>:"OUINON.vi"("errin"=w453, "image"="Montage" ("IN")) -> ("error out"=w452:errorcluster, "OUI/NON"=w448:bool)  [unwired: 8 in]
        n162 = Select ("Sélectionner")(t=w447, s=w448, f=OP300ZP_state."Crash" ("cas faux")) -> (s? t:f=w444:T5)
      }
      frame "Demontage" {
        w458 = OP300ZP_state."Hydrau"  # Énum
        n163 = call <vilib>:"OUINON.vi"("errin"=w462, "image"="Demontage" ("IN")) -> ("error out"=w461:errorcluster, "OUI/NON"=w459:bool)  [unwired: 8 in]
        n164 = Select ("Sélectionner")(t=w458, s=w459, f=OP300ZP_state."Crash" ("cas faux")) -> (s? t:f=w455:T5)
        n165 = local write "TOP"("Demontage du pack" ("TOP")) -> ()
      }
      frame "Crash" {
        # "\\\\forseepower.com\\fr\\040 Production\\FR7 - Poitiers\\06 Production\\05. Electronique\\Documents Control lib\\Archives\\ZEN PLUS"
        n166 = Close File(refnum=w491, error in=w490) -> (path=w478:path, error out=w483:errorcluster)
        n167 = call <vilib>:"waitXms.vi"("attente (ms)"=u32 300, "errin"=w483) -> ("errout"=w479:errorcluster)  [unwired: 13 in]
        n168 = local read "Cluster"() -> (w472:T1)
        n169 = Read from Text File(file (use dialog)=w478, error in=w479) -> (text=w477:string, error out=w475:errorcluster)  [unwired: 2 in, 2 out]
        n170 = call "OP300ZP_SN_Reader.vi"("Fichier txt"=w477) -> ("SN"=w470:string)  [unwired: 10 in]
        n171 = Unbundle By Name(w472) -> ("PN"=w469:string)
        n172 = call <vilib>:"FGV_Image.vi"("Énum"=FGV."SET", "IN"="TeamLeader") -> ()  [unwired: 9 in, 1 out]
        n173 = Concatenate Strings(w469, "-SN" ("chaîne"), w470) -> (w471:string)
        n174 = call "OP300ZP_NouveauDossier.vi"("entrée d'erreur (pas d'erreur)"=w475, "Nom du repertoire (PN SN)"=w471, "Network before adding a new folder"=path "\\\\forseepower.com\\fr/040 Production/FR7 - Poitiers/06 Production/05. Electronique/Documents Control lib/Archives/ZEN PLUS" ("chemin de la cible (utiliser une boîte de dialogue)")) -> ("sortie d'erreur"=w476:errorcluster, "Network after adding a new folder"=w473:path)  [unwired: 7 in]
        n175 = Copy ("Copier")(8:w476, 10:w473, 11:w478) -> (0:w482:errorcluster)  [unwired: 2 in, 2 out]
        n176 = call "PvgeneratorOP300.vi"("errin"=w482, "network"=w473, "path in"=w478) -> ("sortie d'erreur"=w486:errorcluster, "network out"=w485:path)  [unwired: 5 in, 2 out]
        n177 = call <vilib>:"POP_GOOGLE.vi"("error in"=w486, "chemin"=w485) -> ("error out"=w481:errorcluster)  [unwired: 8 in, 1 out]
        n178 = disable-structure shown="Désactivé" {
          disable-tunnel: w481 -> [w500 _]
          disable-tunnel: [w499 _] -> w480
          frame Disabled {
            n179 = Select ("Sélectionner")(t="1", s=FALSE ("sélecteur"), f="0" ("cas faux")) -> (s? t:f=w495:string)
            n180 = local read "Cluster"() -> (w498:T1)
            n181 = Bundle By Name(cluster=w498, "Résultat final"=w495) -> (w494:T1)
            n182 = call "BDD_2.vi"("errin"=w500, "Cluster"=w494) -> ("error out"=w499:errorcluster)  [unwired: 8 in, 1 out]
          }
          frame Enabled {
          }
        }
        n183 = flat-sequence {
          tunnel: [TRUE] -> w492
          tunnel: w480 -> [_]
          frame #0 {
          }
        }
      }
      frame "Next" {
        w528 = OP300ZP_state."Null"  # Énum
        w529 = OP300ZP_state."Scan"  # Énum
        # "\\\\forseepower.com\\fr\\040 Production\\FR7 - Poitiers\\06 Production\\05. Electronique\\Documents Control lib\\Archives\\ZEN PLUS"
        n184 = Close File(refnum=w531, error in=w530) -> (path=w508:path, error out=w527:errorcluster)
        n185 = call <vilib>:"waitXms.vi"("attente (ms)"=u32 300, "errin"=w527) -> ("errout"=w520:errorcluster)  [unwired: 13 in]
        n186 = local read "Cluster"() -> (w513:T1)
        n187 = Read from Text File(file (use dialog)=w508, error in=w520) -> (text=w518:string, error out=w517:errorcluster)  [unwired: 2 in, 2 out]
        n188 = call "OP300ZP_SN_Reader.vi"("Fichier txt"=w518) -> ("SN"=w510:string)  [unwired: 10 in]
        n189 = Unbundle By Name(w513) -> ("PN"=w512:string)
        n190 = Concatenate Strings(w512, "-SN" ("chaîne"), w510) -> (w509:string)
        n191 = call "Multi_OUI_NON.vi"("errin"=w507, "errinb"=TRUE, "Tableau"=string[] ["SECU", "Next"]) -> ("errout"=w505:errorcluster, "isok?"=w504:bool)  [unwired: 7 in]
        n192 = call "OP300ZP_NouveauDossier.vi"("entrée d'erreur (pas d'erreur)"=w517, "Nom du repertoire (PN SN)"=w509, "Network before adding a new folder"=path "\\\\forseepower.com\\fr/040 Production/FR7 - Poitiers/06 Production/05. Electronique/Documents Control lib/Archives/ZEN PLUS" ("chemin de la cible (utiliser une boîte de dialogue)")) -> ("sortie d'erreur"=w516:errorcluster, "Network after adding a new folder"=w514:path)  [unwired: 7 in]
        n193 = Copy ("Copier")(8:w516, 10:w514, 11:w508) -> (0:w519:errorcluster)  [unwired: 2 in, 2 out]
        n194 = call "PvgeneratorOP300.vi"("errin"=w519, "network"=w514, "path in"=w508) -> ("sortie d'erreur"=w525:errorcluster, "network out"=w524:path, "tout bon"=w521:bool)  [unwired: 5 in, 1 out]
        n195 = call <vilib>:"POP_GOOGLE.vi"("error in"=w525, "chemin"=w524) -> ("error out"=w522:errorcluster)  [unwired: 8 in, 1 out]
        n196 = Select(t=w529, s=w504, f=w528) -> (s? t:f=w502:T5)
        n197 = disable-structure shown="Désactivé" {
          disable-tunnel: [w539 _] -> w523
          disable-tunnel: w522 -> [w538 _]
          disable-tunnel: w521 -> [w536 _]
          frame Disabled {
            n198 = Select ("Sélectionner")(t="1", s=w536, f="0" ("cas faux")) -> (s? t:f=w533:string)
            n199 = local read "Cluster"() -> (w537:T1)
            n200 = Bundle By Name(cluster=w537, "Résultat final"=w533) -> (w532:T1)
            n201 = call "BDD_2.vi"("errin"=w538, "Cluster"=w532) -> ("error out"=w539:errorcluster)  [unwired: 8 in, 1 out]
          }
          frame Enabled {
          }
        }
      }
      frame "Hydrau" {
        n202 = disable-structure shown="Désactivé" {
          disable-tunnel: w547 -> [w568 _]
          disable-tunnel: w546 -> [w567 _]
          disable-tunnel: [w566 _] -> w545
          disable-tunnel: [w565 _] -> w544
          disable-tunnel: [w560 _] -> w542
          disable-tunnel: w541 -> [w557 _]
          disable-tunnel: [w552 _] -> w540
          frame Disabled {
            # "A modifier avec hydrau haut"
            n203 = global write "VG_HYDRAU.vi" "CONTI HYDRAU"(0.0 ("R")) -> ()
            n204 = call <vilib>:"OUINON.vi"("errin"=w557, "image"="CONTI_HYDRAU" ("IN")) -> ("error out"=w549:errorcluster, "OUI/NON"=w555:bool)  [unwired: 8 in]
            n205 = global read "VG_BT3562.vi" "BT3562"() -> (w548:string)
            n206 = local write "TOP"("Continuité Blocs hydrauliques haut" ("TOP")) -> ()
            n207 = flat-sequence {
              tunnel: w555 -> [w573]
              tunnel: [w572] -> w569
              tunnel: w549 -> [w571]
              tunnel: w548 -> [w570]
              tunnel: [w608] -> w550
              tunnel: [w607] -> w554
              tunnel: [w606] -> w553
              tunnel: w569 -> [w606]
              frame #0 {
                n208 = case shown="Vrai" w573 {
                  tunnel: [w574 w578] -> w572
                  tunnel: w571 -> [w574 w576]
                  tunnel: w570 -> [_ w575]
                  frame False {
                  }
                  frame True {
                    n209 = while {
                      tunnel: [w590] -> w577
                      tunnel: w576 -> [w581]
                      tunnel: w575 -> [w580]
                      i -> [w589]
                      stop <- w586 stop-if-true
                      n210 = local read "VISA OUT"() -> (w582:T2)
                      n211 = call <vilib>:"Application Directory.vi"() -> ("Application Directory"=w592:path)
                      n212 = Unbundle By Name(w582) -> ("3562"=w584:string)
                      n213 = global read "VG_HYDRAU.vi" "CONTI HYDRAU"() -> (w583:dbl)
                      n214 = call <userlib>:"ACIR_DCIR_BT3562.vi"("errin"=w581, "chemin de base"=w592, "section"=w584, "VISAin"=w580) -> ("errout"=w585:errorcluster, "R pass"=w591:bool, "R Out float"=w587:dbl)  [unwired: 1 in, 4 out]
                      n215 = Greater Or Equal?(x=w587, y=w583) -> (x >= y?=w588:bool)
                      n216 = case shown="Vrai" w591 {
                        selector: w591 -> [w595 _]
                        tunnel: w585 -> [w593 w597]
                        tunnel: [w593 w599] -> w590
                        tunnel: [w594 "last?"] -> w586
                        tunnel: w589 -> [_ w602]
                        frame False {
                          n217 = Not(x=w595) -> (.not. x?=w594:bool)
                        }
                        frame True {
                          n218 = Add(x=1, y=w602) -> ()  [unwired: 1 out]
                          n219 = call <vilib>:"FGV_Image.vi"("Énum"=FGV."SET", "IN"="2ndBloc") -> ()  [unwired: 9 in, 1 out]
                          n220 = property on="last?" class="Bool"(error in=w597, "Visible"=TRUE) -> (error out=w599:errorcluster)  [unwired: 1 in, 1 out]
                          n221 = Wait (ms)(milliseconds to wait=u32 4000 ("attente (ms)")) -> ()  [unwired: 1 out]
                        }
                      }
                      n222 = case shown="Vrai" w588 {
                        tunnel: w587 -> [_ w605]
                        frame False {
                        }
                        frame True {
                          n223 = global write "VG_HYDRAU.vi" "CONTI HYDRAU"(w605) -> ()
                        }
                      }
                    }
                    n224 = property on="last?" class="Bool"(error in=w577, "Visible"=FALSE) -> (error out=w578:errorcluster)  [unwired: 1 in, 1 out]
                  }
                }
              }
              frame #1 {
                n225 = call <vilib>:"Application Directory.vi"() -> ("Application Directory"=w612:path)
                n226 = global read "VG_HYDRAU.vi" "CONTI HYDRAU"() -> (w607:dbl)
                n227 = call "Read_Param.vi"("Énum"=enum16{"STR", "DBL", "U32"}."DBL", 9:w612, "section"="Conti", "key"="Rmax") -> ("dbl"=w610:dbl)  [unwired: 3 in, 4 out]
                n228 = In Range and Coerce(upper limit=w610, x=w607, lower limit=1.0 ("limite inférieure")) -> (In Range?=w608:bool)  [unwired: 1 out]
              }
            }
            n229 = case shown="Vrai" w550 {
              tunnel: w568 -> [w615 w623]
              tunnel: w567 -> [w617 w622]
              tunnel: [w617 w621] -> w566
              tunnel: ["0" w620] -> w561
              tunnel: [w615 w619] -> w560
              tunnel: w554 -> [_ w618]
              frame False {
              }
              frame True {
                n230 = Number To Decimal String(number=w618) -> (decimal integer string=w620:string)  [unwired: 1 in]
                n231 = Concatenate Strings("Hydrau;" ("chaîne"), w620) -> (w625:string)
                n232 = call <vilib>:"Log_basic.vi"("errin"=w623, "date?"=TRUE, "chaîne"=w625, "in"=w622) -> ("sortie d'erreur"=w619:errorcluster, "refnum en sortie"=w621:refnum<file>)  [unwired: 6 in]
              }
            }
            n233 = local read "Cluster"() -> (w563:T1)
            n234 = Bundle By Name(cluster=w563, "Sealing"=w561) -> (w562:T1)
            n235 = call "ZenPlusOP300_refaire.vi"("refaire"=OP300ZP_state."Hydrau" ("Cas OK"), "casOK"=OP300ZP_state."Sealing" ("Cas OK"), "errin"=w553, "test ok ?"=w550) -> ("errout"=w565:errorcluster, "Next"=w552:T5)  [unwired: 6 in]
            n236 = local write "Cluster"(w562) -> ()
          }
          frame Enabled {
          }
        }
      }
      frame "Sealing" {
        n237 = call "OP300ZP_SEALING.vi"("ERRIN"=w644) -> ("ERROUT"=w628:errorcluster, "SEALING_VALUE"=w640:dbl, "IsOK?"=w630:bool)  [unwired: 8 in]
        n238 = case shown="Vrai" w630 {
          tunnel: [FALSE ("OUI/NON") w649] -> w629
          tunnel: w628 -> [w645 w648]
          tunnel: [w645 w647] -> w627
          frame False {
          }
          frame True {
            n239 = call <vilib>:"OUINON.vi"("errin"=w648, "image"="VERIF" ("IN")) -> ("error out"=w647:errorcluster, "OUI/NON"=w649:bool)  [unwired: 8 in]
          }
        }
        n240 = call "ZenPlusOP300_refaire.vi"("refaire"=w633, "casOK"=OP300ZP_state."Next" ("Cas OK"), "errin"=w627, "test ok ?"=w629) -> ("errout"=w631:errorcluster, "Next"=w632:T5)  [unwired: 6 in]
        n241 = case shown="Vrai" w630 {
          tunnel: w639 -> [w651 w659]
          tunnel: w637 -> [w653 w658]
          tunnel: [w653 w657] -> w636
          tunnel: ["0" w656] -> w641
          tunnel: [w651 w655] -> w638
          tunnel: w640 -> [_ w654]
          frame False {
          }
          frame True {
            n242 = Number To Decimal String(number=w654) -> (decimal integer string=w656:string)  [unwired: 1 in]
            n243 = Concatenate Strings("Sealing;" ("chaîne"), w656) -> (w661:string)
            n244 = call <vilib>:"Log_basic.vi"("errin"=w659, "date?"=TRUE, "chaîne"=w661, "in"=w658) -> ("sortie d'erreur"=w655:errorcluster, "refnum en sortie"=w657:refnum<file>)  [unwired: 6 in]
          }
        }
        n245 = local read "Cluster"() -> (w643:T1)
        n246 = Bundle By Name(cluster=w643, "Sealing"=w641) -> (w642:T1)
        n247 = local write "Cluster"(w642) -> ()
      }
      frame "Comext" {
        n248 = disable-structure shown="Activé" {
          disable-tunnel: w672 -> [w685 _]
          disable-tunnel: w671 -> [w684 _]
          disable-tunnel: [w683 _] -> w670
          disable-tunnel: [w682 _] -> w669
          disable-tunnel: w668 -> [w681 _]
          disable-tunnel: [w680 _] -> w667
          disable-tunnel: w666 -> [w678 _]
          disable-tunnel: [w676 _] -> w665
          disable-tunnel: w664 -> [w675 _]
          disable-tunnel: [w673 _] -> w663
          frame Disabled {
            n249 = call <vilib>:"OUINON.vi"("errin"=w678, "image"="Comext" ("IN")) -> ("error out"=w677:errorcluster, "OUI/NON"=w674:bool)  [unwired: 8 in]
            n250 = case shown="Vrai" w674 {
              tunnel: w685 -> [w690 w701]
              tunnel: w684 -> [w689 w700]
              tunnel: [w689 w699] -> w683
              tunnel: [w690 w698] -> w682
              tunnel: [OP300ZP_state."Crash" ("OUT") w697] -> w673
              tunnel: w681 -> [_ w696]
              tunnel: [w687 w691] -> w680
              tunnel: w677 -> [w687 w695]
              tunnel: [w688 w694] -> w676
              tunnel: w675 -> [w688 w694]
              frame False {
              }
              frame True {
                (unwired) u8 0 ("progression")
                (unwired) FALSE ("Visible")
                (unwired) u8 0 ("progression")
                (unwired) TRUE ("Visible")
                w707 = OP300ZP_state."Demontage"  # Énum
                n251 = local read "PN"() -> (w705:string)
                n252 = call "Read_Param.vi"("Énum"=enum16{"STR", "DBL", "U32"}."U32", "errin"=w695, "section"="DataDyn", "key"=w705) -> ("U32"=w703:u32)  [unwired: 3 in, 4 out]
                n253 = call <vilib>:"FGV_Image.vi"("Énum"=FGV."SET", "IN"="DataDyn") -> ()  [unwired: 9 in, 1 out]
                n254 = call "SCAN CMU.vi"("Nb modules"=w703) -> ("errout"=w716:errorcluster, "# température + #tension OK?"=w711:bool, "Vmin"=w715:dbl, "Vmax"=w714:dbl, "Tmin"=w712:dbl, "Tmax"=w713:dbl)  [unwired: 1 in, 4 out]
                n255 = call "OP300ZP_Test_DataDyn.vi"("Vcell Max (V)"=w714, "MCU"=w711, "Vcell Min (V)"=w715, "errin"=w716, "Température usine (°C)"=21.0, "Tcell Max (°C)"=w713, "Tcell Min (°C)"=w712) -> ("errout"=w710:errorcluster, "datalog"=w718:string, "pass"=w709:bool)  [unwired: 1 in, 1 out]
                n256 = call <vilib>:"Log_basic.vi"("errin"=w701, "date?"=TRUE, "chaîne"=w718, "in"=w700) -> ("sortie d'erreur"=w698:errorcluster, "refnum en sortie"=w699:refnum<file>)  [unwired: 6 in]
                n257 = call "ZenPlusOP300_refaire.vi"("refaire"=w696, "Pédale"=FALSE, "casOK"=w707, "errin"=w710, "test ok ?"=w709) -> ("errout"=w691:errorcluster, "Next"=w697:T5)  [unwired: 5 in]
              }
            }
          }
          frame Enabled {
            n258 = One Button Dialog(message="ERR0897") -> ()  [unwired: 1 in, 1 out]
          }
        }
      }
      frame "OCV" {
        w742 = enum16{"STR", "DBL", "U32"}."DBL" ("Énum")
        n259 = call "Multi_OUI_NON.vi"("errin"=w755, "errinb"=TRUE, "Tableau"=string[] ["ISOMAN1", "ISOMAN2", "ISOMAN3"]) -> ("errout"=w735:errorcluster, "isok?"=w732:bool)  [unwired: 7 in]
        n260 = global read "VG_MX5060.vi" "MX5060"() -> (w729:string)
        n261 = case shown="Vrai" w732 {
          tunnel: [0.0 ("Vout lissée") w775] -> w756
          tunnel: w735 -> [w770 w774]
          tunnel: [w770 w773] -> w733
          tunnel: w729 -> [_ w772]
          frame False {
          }
          frame True {
            n262 = call "OP300ZP_Vout.vi"("errin"=w774, "VISA"=w772) -> ("errout"=w773:errorcluster, "Vout lissée"=w775:dbl)  [unwired: 8 in]
          }
        }
        n263 = global read "IS30%.vi" "VG IS30% ?"() -> (w736:bool)
        n264 = Select ("Sélectionner")(t="OCV30" ("section"), s=w736, f="OCV70" ("cas faux")) -> (s? t:f=w737:string)
        n265 = local write "TOP"("Mesure de l'OCV" ("TOP")) -> ()
        n266 = call "Read_Param.vi"("Énum"=w742, "errin"=w733, "section"=w737, "key"="OCVmax") -> ("error out"=w743:errorcluster, "dbl"=w741:dbl)  [unwired: 3 in, 3 out]
        n267 = call "Read_Param.vi"("Énum"=w742, "errin"=w743, "section"=w737, "key"="OCVmin") -> ("error out"=w754:errorcluster, "dbl"=w740:dbl)  [unwired: 3 in, 3 out]
        n268 = In Range and Coerce(upper limit=w741, x=w756, lower limit=w740) -> (In Range?=w730:bool)  [unwired: 1 out]
        n269 = case shown="Vrai" w730 {
          tunnel: w754 -> [w779 w809]
          tunnel: [w776 w807] -> w727
          tunnel: [w776 w784] -> w728
          tunnel: [w780 w806] -> w753
          tunnel: [w780 w805] -> w752
          tunnel: [w779 w796] -> w750
          tunnel: [0.0 ("dbl") w799] -> w751
          tunnel: [FALSE ("OUI/NON") w794] -> w749
          tunnel: [w776 w781] -> w726
          frame False {
            w780 = 0.0 ("DATA FINAL FLT")
            w776 = "" ("DATA FINALE")
          }
          frame True {
            # "Test ISO"
            n270 = call <vilib>:"OUINON.vi"("errin"=w809, "image"="ISOMAN4") -> ("error out"=w793:errorcluster, "OUI/NON"=w808:bool)  [unwired: 8 in]
            n271 = local write "TOP"("Mesure de l'isolement" ("TOP")) -> ()
            n272 = property on="progression" class="Gliss (strict)"(error in=w793, "Visible"=w808, "Value"=u8 0 ("progression")) -> ()  [unwired: 1 in, 2 out]
            n273 = global read "VG_ST5520.vi" "ST5520"() -> (w782:string)
            n274 = call "ST5520_CMD.vi"("errin"=w793, "VISA"=w782) -> ("errout"=w783:errorcluster, "DATA FINAL FLT"=w806:dbl, "DATA OUT"=w807:string, "60s?"=w798:bool)  [unwired: 6 in]
            n275 = property on="progression" class="Gliss (strict)"(error in=w783, "Visible"=FALSE, "Value"=u8 0 ("progression")) -> ()  [unwired: 1 in, 2 out]
            n276 = case shown="Vrai" w798 {
              tunnel: w783 -> [w813 w816]
              tunnel: [w813 w815] -> w791
              tunnel: [FALSE ("OUI/NON") w814] -> w789
              frame False {
              }
              frame True {
                n277 = call <vilib>:"OUINON.vi"("errin"=w816, "image"="ISOMAN5") -> ("error out"=w815:errorcluster, "OUI/NON"=w814:bool)  [unwired: 8 in]
              }
            }
            n278 = property on="progression" class="Gliss (strict)"(error in=w791, "Visible"=w789, "Value"=u8 0 ("progression")) -> ()  [unwired: 1 in, 2 out]
            n279 = case shown="Vrai" w789 {
              tunnel: [w818 w822] -> w784
              tunnel: [0.0 ("DATA FINAL FLT") w826] -> w805
              tunnel: [w819 w825] -> w788
              tunnel: w782 -> [_ w824]
              tunnel: w791 -> [w819 w823]
              tunnel: [w818 w821] -> w781
              frame False {
                w818 = "" ("DATA FINALE")
              }
              frame True {
                n280 = call "ST5520_CMD_2.vi"("errin"=w823, "VISA"=w824) -> ("errout"=w825:errorcluster, "DATA FINAL FLT"=w826:dbl, "DATAOUT"=w822:string, "read buffer"=w821:string)  [unwired: 5 in, 1 out]
              }
            }
            n281 = call <vilib>:"Application Directory.vi"() -> ("Application Directory"=w802:path)
            n282 = property on="progression" class="Gliss (strict)"(error in=w788, "Visible"=FALSE, "Value"=u8 0 ("progression")) -> ()  [unwired: 1 in, 2 out]
            n283 = call "Read_Param.vi"("Énum"=enum16{"STR", "DBL", "U32"}."DBL", "errin"=w788, 9:w802, "section"="Iso", "key"="Min") -> ("error out"=w797:errorcluster, "dbl"=w799:dbl)  [unwired: 2 in, 3 out]
            n284 = call <vilib>:"OUINON.vi"("errin"=w797, "image"="ISOMAN6") -> ("error out"=w796:errorcluster, "OUI/NON"=w794:bool)  [unwired: 8 in]
          }
        }
        "ISO-" <- w727
        "ISO+" <- w728
        "ISO- avant découpage" <- w726
        n285 = Number To Fractional String(number=w756, precision (6)=i16 2 ("précision (6)")) -> (F-format string=w759:string)  [unwired: 2 in]
        n286 = Concatenate Strings("OCV;" ("chaîne"), w759, ";ISO+;" ("chaîne"), w727, ";ISO-;" ("chaîne"), w728) -> (w724:string)
        n287 = call <vilib>:"Log_basic.vi"("errin"=w766, "date?"=TRUE, "chaîne"=w724, "in"=w768) -> ("sortie d'erreur"=w765:errorcluster, "refnum en sortie"=w764:refnum<file>)  [unwired: 6 in]
        n288 = local read "Cluster"() -> (w761:T1)
        n289 = Bundle By Name(cluster=w761, "OCV"=w759, "ISOP"=w727, "ISOM"=w728) -> (w760:T1)
        n290 = local write "Cluster"(w760) -> ()
        n291 = Greater?(x=w752, y=w751) -> (0:w747:bool)
        n292 = Greater?(x=w753, y=w751) -> (0:w748:bool)
        n293 = Compound Arithmetic op=AND ("Opérateur arithmétique")(w749, w748, w747) -> (w746:bool)
        n294 = call "ZenPlusOP300_refaire.vi"("refaire"=w758, "casOK"=OP300ZP_state."DataDyn" ("Cas OK"), "errin"=w750, "test ok ?"=w746) -> ("errout"=w763:errorcluster, "Next"=w757:T5)  [unwired: 6 in]
      }
    }
    n295 = Wait (ms)(milliseconds to wait=u32 200 ("attente (ms)")) -> ()  [unwired: 1 out]
    n296 = case shown="Faux" w21 {
      selector: w21 -> [_ w28]
      frame False {
      }
      frame True {
        n297 = local write "STOP"(w28) -> ()
      }
    }
  }
  n298 = while {
    shift-right: [w835] -> _
    shift-left: errorcluster {"status"=FALSE, "code"=0, "source"=""} ("error out") -> [w832]
    stop <- w833 stop-if-true
    # "ici tu met l'image à jour si besoin"
    n299 = Wait (ms)(milliseconds to wait=u32 10 ("attente (ms)")) -> ()  [unwired: 1 out]
    n300 = call <vilib>:"FGV_Image.vi"("Énum"=FGV."GET") -> ("OUT"=w828:string)  [unwired: 10 in]
    n301 = Not Equal?(x=w828, y="") -> (x != y?=w829:bool)
    n302 = case shown="Faux" w829 {
      tunnel: [w837 w842] -> w835
      tunnel: w832 -> [w837 w841]
      tunnel: w828 -> [_ w840]
      frame False {
      }
      frame True {
        n303 = call <vilib>:"Application Directory.vi"() -> ("Application Directory"=w845:path)
        n304 = Path To String(path=w845) -> (string=w846:string)
        n305 = Concatenate Strings(w846, "\\Image\\" ("chaîne"), w840, ".jpg" ("chaîne")) -> (w844:string)
        n306 = call <vilib>:"FGV_Image.vi"("Énum"=FGV."RAZ") -> ()  [unwired: 10 in, 1 out]
        n307 = String To Path(string=w844) -> (path=w843:path)
        n308 = call <vilib>:"Read JPEG File.vi"("error in (no error)"=w841, "path to JPEG file"=w843) -> ("error out"=w842:errorcluster, "image data"=w849:T9)  [unwired: 7 in, 1 out]
        n309 = call <vilib>:"Draw Flattened Pixmap.vi"("image data"=w849) -> ("new picture"=w838:picture)  [unwired: 8 in]
        n310 = local write "DRAW"(w838) -> ()
      }
    }
    n311 = global read "VG_progressBar.vi" "progression"() -> (→"progression":dbl)
    n312 = local read "STOP"() -> (w834:bool)
    n313 = Or(x=w835, y=w834) -> (x .or. y?=w833:bool)
  }
  n314 = Merge Errors(w14, w13) -> (→"errout":errorcluster)
  n315 = disable-structure shown="Activé" {
    disable-tunnel: [w850 _] -> _
    frame Disabled {
      n316 = call "Data Dynamiques"() -> ("CMU OK"=w850:bool)  [unwired: 12 in, 7 out]
    }
    frame Enabled {
    }
  }
  "STOP" <- w11
